vi "firebase_array_maker.vi"(10 "be_string":string) -> (0 "indexek_ nevei":string[](array[string]), 3 "json ki":string)   [LabVIEW 2015]
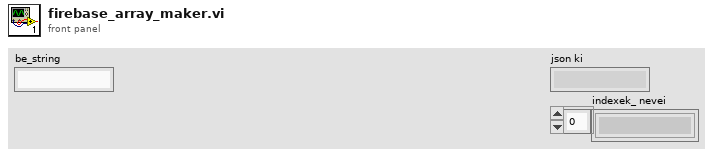
[diagram p1: front panel]
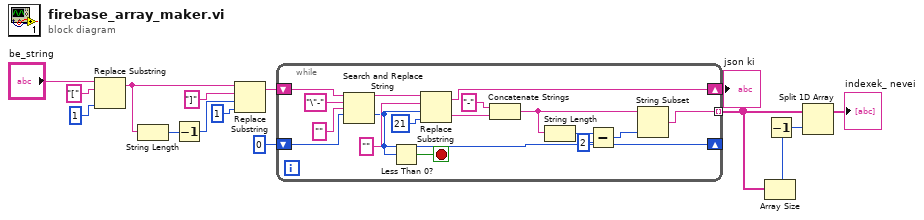
[diagram p0: block diagram]
diagram:
  n1 = Replace Substring(2:1 ("length (len. of substring)"), 4:"[" ("substring (\"\")"), 5:"be_string") -> (1:w10:string)  [unwired: 1 in, 1 out]
  n2 = String Length(string=w10) -> (length=w13:i32)
  n3 = Decrement(x=w13) -> (x-1=w12:i32)
  n4 = Replace Substring(2:1 ("length (len. of substring)"), 3:w12, 4:"]" ("substring (\"\")"), 5:w10) -> (1:w8:string)  [unwired: 1 out]
  n5 = while {
    shift-right: [w31] -> w5
    shift-left: w8 -> [w32]
    shift-right: [w23] -> _
    shift-left: 0 ("offset past replacement") -> [w25]
    tunnel: [w16] -> w1 mode=indexing
    stop <- w24 stop-if-true
    n6 = Search and Replace String(input string=w32, search string="\"-", replace string="" ("replace string (\"\")"), offset=w25) -> (result string=w29:string, offset past replacement=w23:i32)  [unwired: 4 in, 2 out]
    n7 = Less Than 0?(x=w23) -> (x < 0?=w24:bool)
    n8 = Replace Substring(2:21 ("length (len. of substring)"), 3:w23, 4:"" ("substring (\"\")"), 5:w29) -> (0:w22:string, 1:w31:string)
    n9 = Concatenate Strings("-" ("string"), w22) -> (w20:string)
    n10 = String Length(string=w20) -> (length=w19:i32)
    n11 = Subtract(x=w19, y=2) -> (x-y=w17:i32)
    n12 = String Subset(string=w20, length (rest)=w17) -> (substring=w16:string)  [unwired: 1 in]
  }
  "json ki" <- w5
  n13 = Array Size(array=w1) -> (size(s)=w3:i32)
  n14 = Decrement(x=w3) -> (x-1=w4:i32)
  n15 = Split 1D Array(array=w1, index=w4) -> (first subarray=→"indexek_ nevei":string[])  [unwired: 1 out]
